vi "GaussianFitTruncated.vi"(4 "Array":dbl[](array[numeric]) format="%.2f", 5 "Width":i32) -> (0 "FWHM":dbl format="%.2f", 1 "Maximum":dbl format="%.2f", 2 "Position":dbl format="%.2f")   [LabVIEW 2009]
uses:
  <vilib>/Analysis/NI_AALBase.lvlib
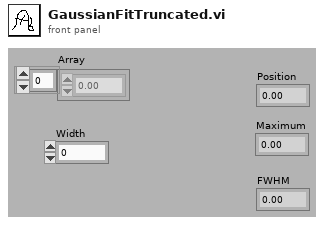
[diagram p1: front panel]
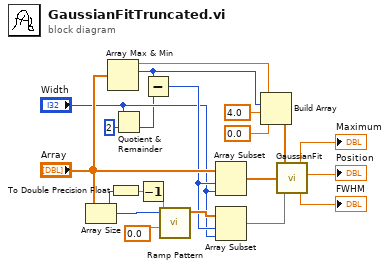
[diagram p0: block diagram]
diagram:
  n1 = Array Size(array="Array") -> (size(s)=w15:i32)
  n2 = Array Max & Min(array="Array") -> (max value=w8:dbl, max index (indices)=w6:i32)  [unwired: 2 out]
  n3 = To Double Precision Float(number=w15) -> (double precision float=w16:dbl)
  n4 = Quotient & Remainder(x="Width", y=2) -> (floor(x/y)=w7:i32)  [unwired: 1 out]
  n5 = Decrement(x=w16) -> (x-1=w17:dbl)
  n6 = Subtract(x=w6, y=w7) -> (x-y=w13:i32)
  n7 = call <vilib>:"Ramp Pattern.vi"("start"=0.0, "end"=w17, "samples"=w15) -> ("Ramp Pattern"=w14:dbl[])  [unwired: 7 in, 1 out]
  n8 = Array Subset(array="Array", index=w13, length="Width") -> (w10:dbl[])
  n9 = Array Subset(array=w14, index=w13, length="Width") -> (w11:dbl[])
  n10 = Build Array(w8, w6, 4.0 ("Elément d'entrée"), 0.0 ("Elément d'entrée")) -> (w9:dbl[])
  n11 = call "GaussianFit.vi"("Initial guess coefficients"=w9, "Input gaussian"=w10, "Input abscissae"=w11) -> ("Amplitude"=→"Maximum":dbl, "Central abscissa"=→"Position":dbl, "FWHM"=→"FWHM":dbl)  [unwired: 1 out]
